vi "Add Only Empty States to Queue Performance Test.vi"() -> ()   [LabVIEW 2020]
panel:
  out "% Improvement":dbl format="%#.1f"
  out "New":u32
  out "Old":u32
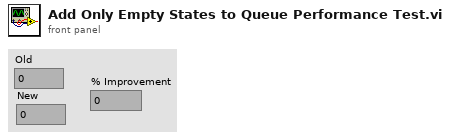
[diagram p1: front panel]
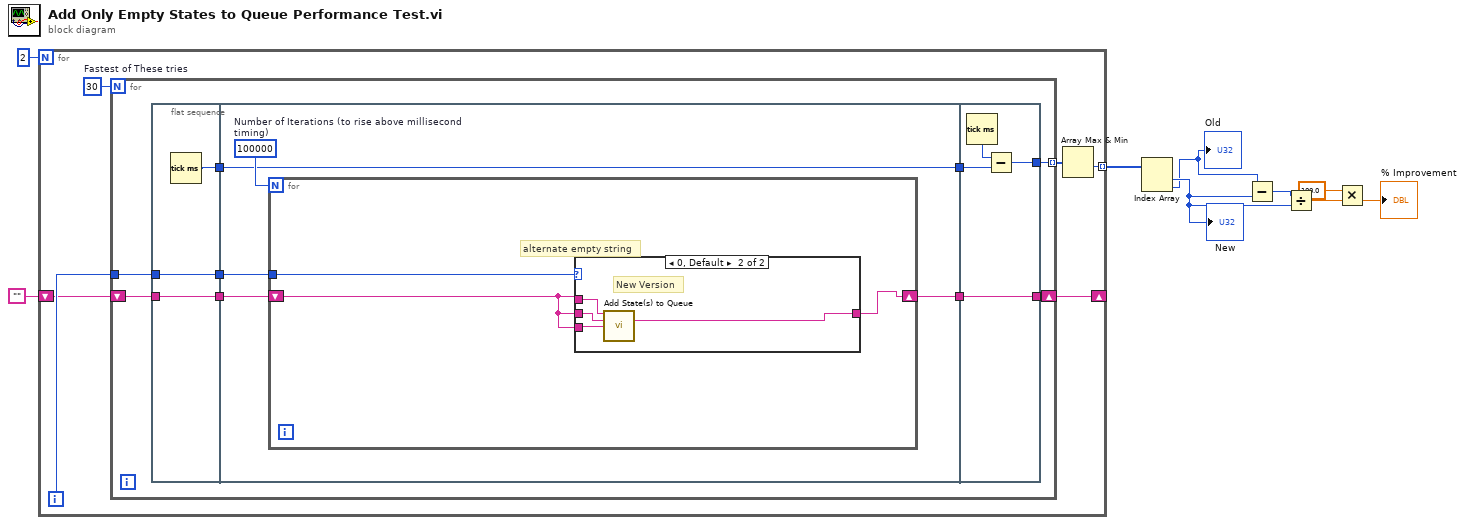
[diagram p0: block diagram]
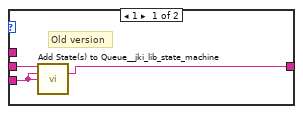
[diagram p2: hidden frame]
diagram:
  n1 = for {
    N: 2 -> [_]
    tunnel: [w12] -> w8 mode=indexing
    shift-right: [w10] -> _
    shift-left: "" -> [w11]
    i -> [w15]
    w13 = 30  # Fastest of These tries
    n2 = for {
      N: w13 -> [_]
      tunnel: w15 -> [w21]
      tunnel: [w20] -> w14 mode=indexing
      shift-right: [w17] -> w10
      shift-left: w11 -> [w18]
      n3 = flat-sequence {
        tunnel: [w27] -> w24
        tunnel: w21 -> [w26]
        tunnel: [w26] -> w23
        tunnel: [w25] -> w19
        tunnel: w18 -> [w25]
        tunnel: w24 -> [w31]
        tunnel: [w31] -> w22
        tunnel: w23 -> [w30]
        tunnel: w19 -> [w29]
        tunnel: [w28] -> w16
        tunnel: w22 -> [w45]
        tunnel: [w44] -> w20
        tunnel: [w43] -> w17
        tunnel: w16 -> [w43]
        frame #0 {
          n4 = Tick Count (ms)() -> (millisecond timer value=w27:u32)
        }
        frame #1 {
          w32 = 100000  # Number of Iterations (to rise above millisecond timing)
          n5 = for {
            N: w32 -> [_]
            tunnel: w30 -> [w35]
            shift-right: [w33] -> w28
            shift-left: w29 -> [w34]
            # "alternate empty string"
            n6 = case shown="0, Default" w35 {
              tunnel: w34 -> [w38 w40]
              tunnel: [w37 w42] -> w33
              tunnel: w34 -> [w36 w41]
              tunnel: w34 -> [_ w39]
              frame 1 {
                # "Old version"
                n7 = call <vilib>:"Add State(s) to Queue__jki_lib_state_machine.vi"("State(s) in Front (\"\")"=w38, "State(s) in (\"\")"=w36, "State(s) at Back (\"\")"=w36) -> ("States Out"=w37:string)  [unwired: 12 in]
              }
              frame 0, Default {
                # "New Version"
                n8 = call "Add State(s) to Queue.vi"("State(s) in Front (\"\")"=w39, "State(s) in (\"\")"=w40, "State(s) at Back (\"\")"=w41) -> ("States Out"=w42:string)  [unwired: 12 in]
              }
            }
          }
        }
        frame #2 {
          n9 = Tick Count (ms)() -> (millisecond timer value=w46:u32)
          n10 = Subtract(x=w46, y=w45) -> (x-y=w44:u32)
        }
      }
    }
    n11 = Array Max & Min(array=w14) -> (min value=w12:u32)  [unwired: 3 out]
  }
  n12 = Index Array(array=w8) -> (element #1=w3:u32, element #2=w2:u32)  [unwired: 2 in]
  "Old" <- w2
  "New" <- w3
  n13 = Subtract(x=w2, y=w3) -> (x-y=w7:u32)
  n14 = Divide(x=w7, y=w3) -> (x/y=w6:dbl)
  n15 = Multiply(x=100.0, y=w6) -> (x*y=→"% Improvement":dbl)
